vi "WSVCAP SHL FPGA LL Procedure RFFE - Send Data.vi"(0 "Procedure Step":T1, 1 "Wait Ticks Remaining":u32, 2 "CMD Length [1-48]":u8, 5 "RFFE Wait Ticks":u32, 7 "Write Bit Index [0-47]":u8, 9 "RFFE Cycle Mode":bool, 11 "error in (no error)":errorcluster, 12 "RFFE Cycle CMD":u64, 13 "Socket Mask":u64) -> (3 "Wait Ticks Remaining Out":u32, 4 "Procedure Step Out":T1, 8 "Write Bit Index [0-47] Out":u8, 10 "Finished":bool, 15 "error out":errorcluster)   [LabVIEW 2012]
uses:
  Type Defs/WSVCAP SHL Procedure Step Enum.ctl
  Type Defs/WSVCAP SHL RFFE Write Line Enum.ctl
  Type Defs/WSVCAP SHL FIFO Operation Enum.ctl
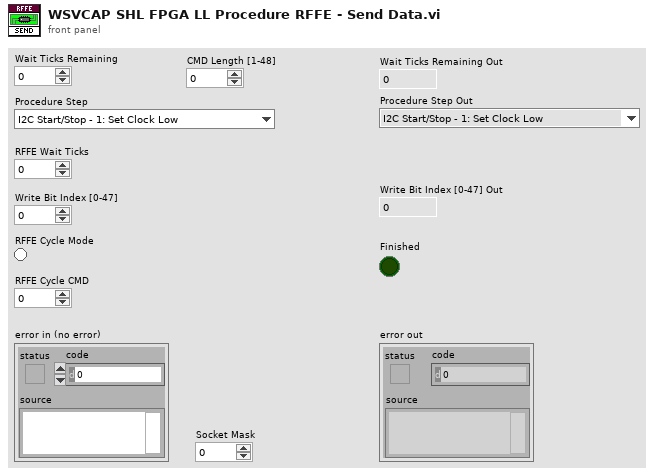
[diagram p1: front panel]
types:
  T1 = typedef "WSVCAP SHL Procedure Step Enum.ctl" = enum16{"I2C Start/Stop - 1: Set Clock Low", "I2C Start/Stop - 2: Wait", "I2C Start/Stop - 3: Set Data I", "I2C Start/Stop - 4: Wait", "I2C Start/Stop - 5: Set Clock High", "I2C Start/Stop - 6: Wait", "I2C Start/Stop - 7: Set Data II", "I2C Start/Stop - 8: Wait", "I2C Start/Stop - 9: Set Clock Low", "I2C Start/Stop - 10: Wait", "I2C Read ACK - 1: Set Clock High", "I2C Read ACK - 2: Wait", "I2C Read ACK - 3: Read ACK Bit", "I2C Read ACK - 4: Wait", "I2C Read ACK - 5: Set Clock Low", "I2C Read ACK - 6: Wait", "I2C Write ACK - 1: Write ACK Bit", "I2C Write ACK - 2: Wait", "I2C Write ACK - 3: Set Clock High", "I2C Write ACK - 4: Wait", "I2C Write ACK - 5: Set Clock Low", "I2C Write ACK - 6: Wait", "I2C Write ACK - 7: Set Data Low", "I2C Send Add - 1: Reset Bits Remaining", "I2C Send Add - 2: Set Data Bit", "I2C Send Add - 3: Wait", "I2C Send Add - 4: Set Clock High", "I2C Send Add - 5: Wait", "I2C Send Add - 6: Set Clock Low", "I2C Send Add - 7: Wait", "I2C Send Add - 8: Check Bits Remaining", "I2C Send Data - 1: Reset Bits Remaining", "I2C Send Data - 2: Load Write Bit from FIFO", "I2C Send Data - 3: Set Data Bit", "I2C Send Data - 4: Wait", "I2C Send Data - 5: Set Clock High", "I2C Send Data - 6: Wait", "I2C Send Data - 7: Set Clock Low", "I2C Send Data - 8: Wait", "I2C Send Data - 9: Check Bits Remaining", "I2C Receive Data - 1: Reset Bits Remaining", "I2C Receive Data - 2: Wait", "I2C Receive Data - 3: Set Clock High", "I2C Receive Data - 4: Wait", "I2C Receive Data - 5: Read Data Bit", "I2C Receive Data - 6: Wait", "I2C Receive Data - 7: Set Clock Low", "I2C Receive Data - 8: Wait", "I2C Receive Data - 9: Check Bits Remaining", "SPI Clear Lines - 1:Clear", "SPI Send/Receive - 1: Load SDA - Clock Low", "SPI Send/Receive - 2: Wait", "SPI Send/Receive - 3: Load DATO - Clock High", "SPI Send/Receive - 4: Wait", "SPI Wait CMD Delay - 1:Wait", "RFFE Send SSC - 1:Set Low", "RFFE Send SSC - 2:Wait", "RFFE Send SSC - 3:Set SDA High", "RFFE Send SSC - 4:Wait", "RFFE Send SSC - 5:Set SDA Low", "RFFE Send SSC - 6:Wait", "RFFE Send Data - 1:Set SCL High", "RFFE Send Data - 2:Wait", "RFFE Send Data - 3:Set SCL Low", "RFFE Send Data - 4:Wait", "RFFE Send Data - 5:Set SCL High (P)", "RFFE Send Data - 6:Wait", "RFFE Send Data - 7:Set SCL Low (P)", "RFFE Send Data - 8:Wait", "RFFE Send Data - 9:Set SCL High (BP)", "RFFE Send Data - 10:Wait", "RFFE Send Data - 11:Set SCL Low (BP)", "RFFE Send Data - 12:Wait", "RFFE Receive Data - 1:Set SCL High", "RFFE Receive Data - 2:Wait", "RFFE Receive Data - 3:Set SCL Low", "RFFE Receive Data - 4:Wait", "RFFE Receive Data - 5:Set SCL High (BP)", "RFFE Receive Data - 6:Wait", "RFFE Receive Data - 7:Set SCL Low (BP)", "RFFE Receive Data - 8:Wait", "RFFE Wait CMD Delay - 1:Wait", "RFFE Clear Lines - 1:Clear"}
  T2 = typedef "WSVCAP SHL RFFE Write Line Enum.ctl" = enum16{"SDAA", "SCLK"}
  T3 = typedef "WSVCAP SHL FIFO Operation Enum.ctl" = enum16{"Create FIFO/Memory", "Get Write FIFO Status", "Get Read FIFO Status", "Put Element in Write", "Put Element in Read", "Get Element from Write", "Get Element from Read"}
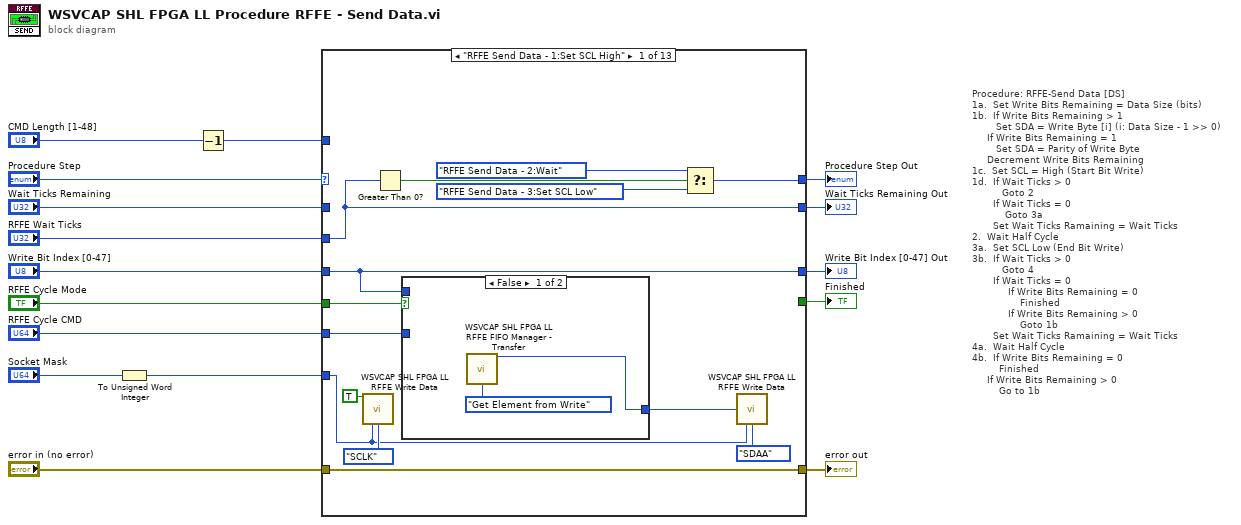
[diagram p0: block diagram]
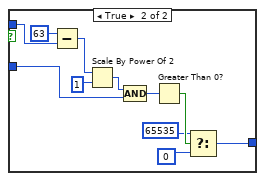
[diagram p2: hidden frame]
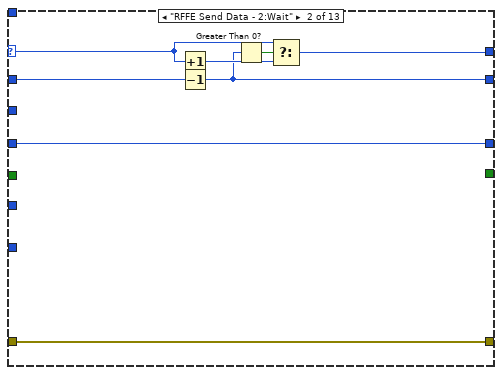
[diagram p3: hidden frame]
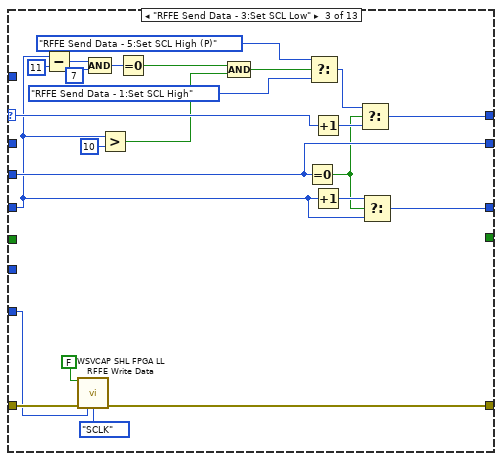
[diagram p4: hidden frame]
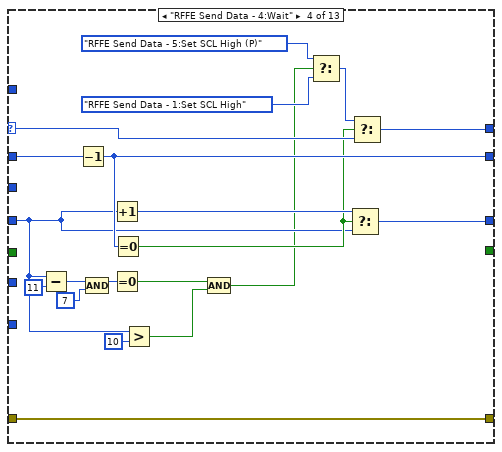
[diagram p5: hidden frame]
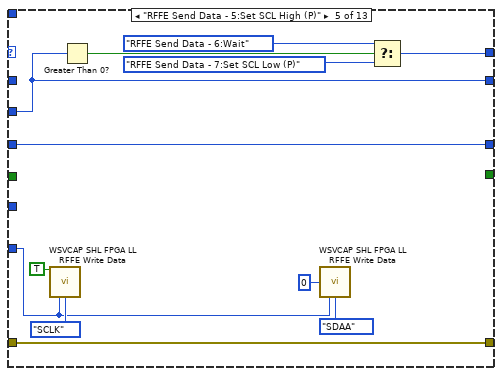
[diagram p6: hidden frame]
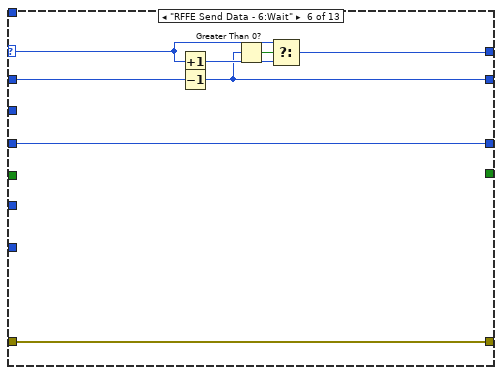
[diagram p7: hidden frame]
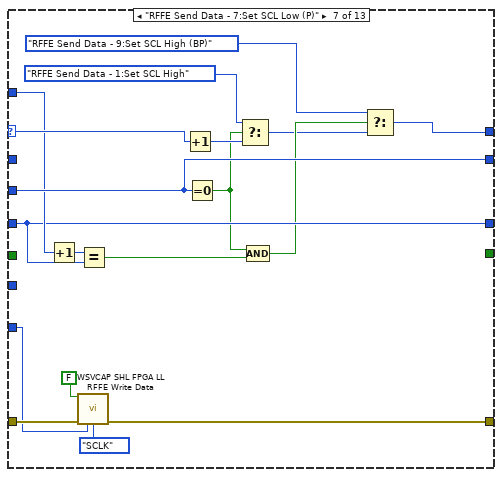
[diagram p8: hidden frame]
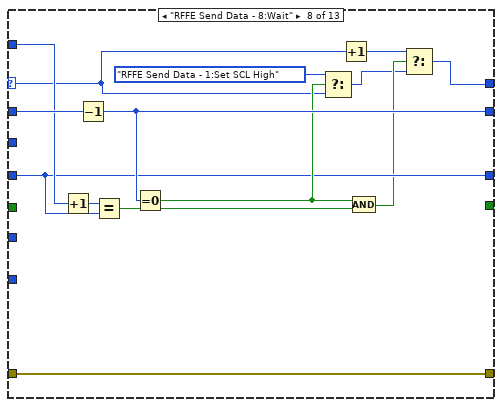
[diagram p9: hidden frame]
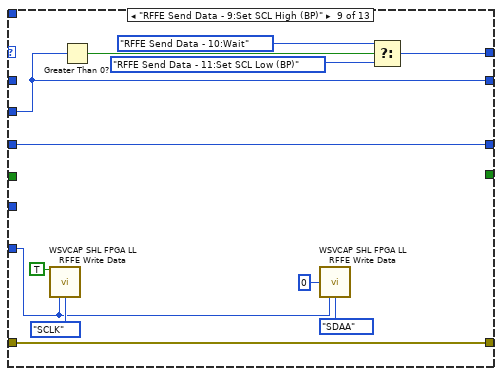
[diagram p10: hidden frame]
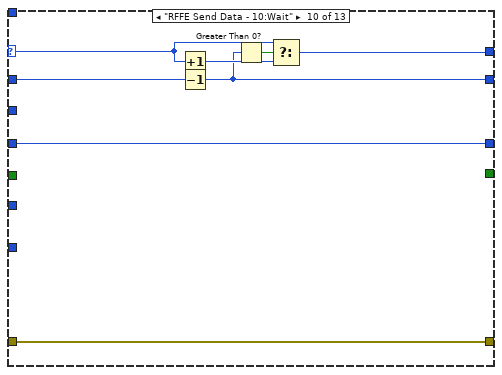
[diagram p11: hidden frame]
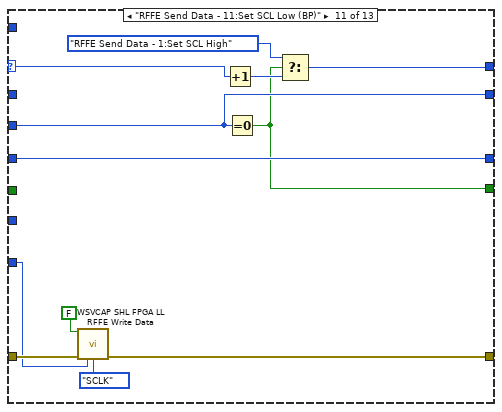
[diagram p12: hidden frame]
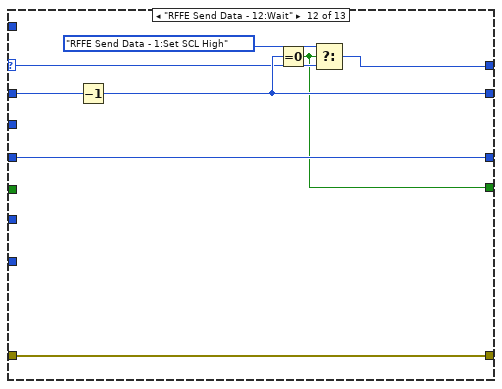
[diagram p13: hidden frame]
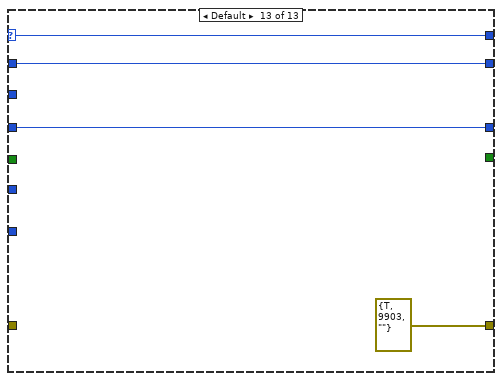
[diagram p14: hidden frame]
diagram:
  # "Procedure: RFFE-Send Data [DS]\n1a.  Set Write Bits Remaining = Data Size (bits)\n1b.  If Write Bits Remaining > 1\n        Set SDA = Write Byte [i] (i: Data Size - 1 >> 0)\n     If Write Bits Remaining = 1\n        Set SDA = Parity of Write Byte\n     Decrement Write Bits Remaining\n1c.  Set SCL = High (Start Bit Write)\n1d.  If Wait Ticks > 0\n          Goto 2\n       If Wait Ticks = 0 \n           Goto 3a\n       Set Wait Ticks Ramaining = Wait Ticks\n2.  Wait Half Cycle\n3a.  Set SCL Low (End Bit Write)\n3b.  If Wait Ticks > 0\n          Goto 4\n       If Wait Ticks = 0 \n            If Write Bits Remaining = 0\n                Finished\n            If Write Bits Remaining > 0\n                Goto 1b\n       Set Wait Ticks Ramaining = Wait Ticks\n4a.  Wait Half Cycle\n4b.  If Write Bits Remaining = 0\n         Finished\n     If Write Bits Remaining > 0\n         Go to 1b"
  n1 = To Unsigned Word Integer(number="Socket Mask") -> (unsigned 16bit integer=w12:u16)
  n2 = Decrement(x="CMD Length [1-48]") -> (x-1=w1:u8)
  n3 = case shown="\"RFFE Send Data - 1:Set SCL High\"" "Procedure Step" {
    selector: "Procedure Step" -> [_ w49 w75 w94 _ w113 w133 w136 _ w165 w179 w182 w190]
    tunnel: [w24 w51 w70 w95 w102 w115 w128 w147 w154 w167 w174 w187 errorcluster {"status"=TRUE, "code"=9903, "source"=""} ("error IO")] -> w15
    tunnel: "error in (no error)" -> [w24 w51 w71 w95 w102 w115 w129 w147 w154 w167 w175 w187 _]
    tunnel: "Wait Ticks Remaining" -> [_ w47 _ w93 _ w111 _ w146 _ w163 _ w186 w189]
    tunnel: "RFFE Wait Ticks" -> [w18 _ w66 _ w98 _ w126 _ w150 _ w171 _ _]
    tunnel: [_ _ _ _ _ _ _ _ _ _ w168 w180 _] -> w14
    tunnel: "Write Bit Index [0-47]" -> [w17 w44 w59 w82 w97 w108 w123 w141 w149 w160 w169 w183 w188]
    tunnel: w12 -> [w26 _ w69 _ w103 _ w127 _ w155 _ w173 _ _]
    tunnel: "RFFE Cycle Mode" -> [w23 _ _ _ _ _ _ _ _ _ _ _ _]
    tunnel: "RFFE Cycle CMD" -> [w22 _ _ _ _ _ _ _ _ _ _ _ _]
    tunnel: w1 -> [_ _ _ _ _ _ w124 w142 _ _ _ _ _]
    tunnel: [w19 w46 w67 w92 w99 w110 w116 w134 w151 w162 w172 w181 w190] -> w5
    tunnel: [w18 w45 w66 w91 w98 w109 w126 w145 w150 w161 w171 w185 w189] -> w4
    tunnel: [w17 w44 w65 w88 w97 w108 w123 w141 w149 w160 w169 w183 w188] -> w3
    frame "RFFE Send Data - 1:Set SCL High" {
      n4 = call "WSVCAP SHL FPGA LL RFFE Write Data.vi"("CLK In"=TRUE ("Bit In"), "Socket Mask"=w26, "Line"=WSVCAP_SHL_RFFE_Write_Line_Enum."SCLK") -> ()  [unwired: 12 in, 1 out]
      n5 = Greater Than 0?(x=w18) -> (x > 0?=w27:bool)
      n6 = case shown="False" w23 {
        tunnel: [w31 w37] -> w25
        tunnel: w22 -> [_ w36]
        tunnel: w17 -> [_ w34]
        frame False {
          n7 = call "WSVCAP SHL FPGA LL RFFE FIFO Manager - Transfer.vi"("Operation"=WSVCAP_SHL_FIFO_Operation_Enum."Get Element from Write") -> ("Data Out"=w31:u16)  [unwired: 12 in, 2 out]
        }
        frame True {
          n8 = Subtract(x=u8 63 ("y"), y=w34) -> (x-y=w33:u8)
          n9 = Scale By Power Of 2(n=w33, x=u64 1 ("Data Out")) -> (x*2^n=w42:u64)
          n10 = Compound Arithmetic op=AND(w42, w36) -> (w41:u64)
          n11 = Greater Than 0?(x=w41) -> (x > 0?=w40:bool)
          n12 = Select(t=u16 65535 ("Data Out"), s=w40, f=u16 0 ("Data Out")) -> (s? t:f=w37:u16)
        }
      }
      n13 = Select(t=WSVCAP_SHL_Procedure_Step_Enum."RFFE Send Data - 2:Wait" ("Procedure Step"), s=w27, f=WSVCAP_SHL_Procedure_Step_Enum."RFFE Send Data - 3:Set SCL Low" ("Procedure Step")) -> (s? t:f=w19:T1)
      n14 = call "WSVCAP SHL FPGA LL RFFE Write Data.vi"("Data Word In"=w25, "Socket Mask"=w26, "Line"=WSVCAP_SHL_RFFE_Write_Line_Enum."SDAA") -> ()  [unwired: 12 in, 1 out]
    }
    frame "RFFE Send Data - 2:Wait" {
      n15 = Increment(x=w49) -> (x+1=w48:T1)
      n16 = Decrement(x=w47) -> (x-1=w45:u32)
      n17 = Greater Than 0?(x=w45) -> (x > 0?=w50:bool)
      n18 = Select(t=w49, s=w50, f=w48) -> (s? t:f=w46:T1)
    }
    frame "RFFE Send Data - 3:Set SCL Low" {
      n19 = Subtract(x=w59, y=u8 11) -> (x-y=w54:u8)
      n20 = call "WSVCAP SHL FPGA LL RFFE Write Data.vi"("CLK In"=FALSE ("Bit In"), "error in (no error)"=w71, "Socket Mask"=w69, "Line"=WSVCAP_SHL_RFFE_Write_Line_Enum."SCLK") -> ("error out"=w70:errorcluster)  [unwired: 11 in]
      n21 = Compound Arithmetic op=AND(w54, u8 7 ("y")) -> (w52:u8)
      n22 = Greater?(x=w59, y=u8 10) -> (0:w56:bool)
      n23 = Equal To 0?(x=w52) -> (x = 0?=w57:bool)
      n24 = Compound Arithmetic op=AND(w57, w56) -> (w55:bool)
      n25 = Equal To 0?(x=w66) -> (x = 0?=w61:bool)
      n26 = Select(t=WSVCAP_SHL_Procedure_Step_Enum."RFFE Send Data - 5:Set SCL High (P)" ("Procedure Step"), s=w55, f=WSVCAP_SHL_Procedure_Step_Enum."RFFE Send Data - 1:Set SCL High" ("Procedure Step")) -> (s? t:f=w62:T1)
      n27 = Increment(x=w75) -> (x+1=w74:T1)
      n28 = Increment(x=w59) -> (x+1=w68:u8)
      n29 = Select(t=w62, s=w61, f=w74) -> (s? t:f=w67:T1)
      n30 = Select(t=w68, s=w61, f=w59) -> (s? t:f=w65:u8)
    }
    frame "RFFE Send Data - 4:Wait" {
      n31 = Subtract(x=w82, y=u8 11) -> (x-y=w78:u8)
      n32 = Decrement(x=w93) -> (x-1=w91:u32)
      n33 = Compound Arithmetic op=AND(w78, u8 7 ("y")) -> (w77:u8)
      n34 = Increment(x=w82) -> (x+1=w90:u8)
      n35 = Equal To 0?(x=w77) -> (x = 0?=w80:bool)
      n36 = Equal To 0?(x=w91) -> (x = 0?=w89:bool)
      n37 = Greater?(x=w82, y=u8 10) -> (0:w81:bool)
      n38 = Compound Arithmetic op=AND(w80, w81) -> (w79:bool)
      n39 = Select(t=WSVCAP_SHL_Procedure_Step_Enum."RFFE Send Data - 5:Set SCL High (P)" ("Procedure Step"), s=w79, f=WSVCAP_SHL_Procedure_Step_Enum."RFFE Send Data - 1:Set SCL High" ("Procedure Step")) -> (s? t:f=w85:T1)
      n40 = Select(t=w90, s=w89, f=w82) -> (s? t:f=w88:u8)
      n41 = Select(t=w85, s=w89, f=w94) -> (s? t:f=w92:T1)
    }
    frame "RFFE Send Data - 5:Set SCL High (P)" {
      n42 = call "WSVCAP SHL FPGA LL RFFE Write Data.vi"("CLK In"=TRUE ("Bit In"), "Socket Mask"=w103, "Line"=WSVCAP_SHL_RFFE_Write_Line_Enum."SCLK") -> ()  [unwired: 12 in, 1 out]
      n43 = Greater Than 0?(x=w98) -> (x > 0?=w104:bool)
      n44 = call "WSVCAP SHL FPGA LL RFFE Write Data.vi"("Data Word In"=u16 0, "Socket Mask"=w103, "Line"=WSVCAP_SHL_RFFE_Write_Line_Enum."SDAA") -> ()  [unwired: 12 in, 1 out]
      n45 = Select(t=WSVCAP_SHL_Procedure_Step_Enum."RFFE Send Data - 6:Wait" ("Procedure Step"), s=w104, f=WSVCAP_SHL_Procedure_Step_Enum."RFFE Send Data - 7:Set SCL Low (P)" ("Procedure Step")) -> (s? t:f=w99:T1)
    }
    frame "RFFE Send Data - 6:Wait" {
      n46 = Increment(x=w113) -> (x+1=w112:T1)
      n47 = Decrement(x=w111) -> (x-1=w109:u32)
      n48 = Greater Than 0?(x=w109) -> (x > 0?=w114:bool)
      n49 = Select(t=w113, s=w114, f=w112) -> (s? t:f=w110:T1)
    }
    frame "RFFE Send Data - 7:Set SCL Low (P)" {
      n50 = Increment(x=w124) -> (x+1=w120:u8)
      n51 = call "WSVCAP SHL FPGA LL RFFE Write Data.vi"("CLK In"=FALSE ("Bit In"), "error in (no error)"=w129, "Socket Mask"=w127, "Line"=WSVCAP_SHL_RFFE_Write_Line_Enum."SCLK") -> ("error out"=w128:errorcluster)  [unwired: 11 in]
      n52 = Equal?(x=w120, y=w123) -> (x = y?=w121:bool)
      n53 = Increment(x=w133) -> (x+1=w132:T1)
      n54 = Equal To 0?(x=w126) -> (x = 0?=w122:bool)
      n55 = Select(t=WSVCAP_SHL_Procedure_Step_Enum."RFFE Send Data - 1:Set SCL High" ("Procedure Step"), s=w122, f=w132) -> (s? t:f=w118:T1)
      n56 = Compound Arithmetic op=AND(w122, w121) -> (w119:bool)
      n57 = Select(t=WSVCAP_SHL_Procedure_Step_Enum."RFFE Send Data - 9:Set SCL High (BP)" ("Procedure Step"), s=w119, f=w118) -> (s? t:f=w116:T1)
    }
    frame "RFFE Send Data - 8:Wait" {
      n58 = Increment(x=w142) -> (x+1=w139:u8)
      n59 = Decrement(x=w146) -> (x-1=w145:u32)
      n60 = Equal?(x=w139, y=w141) -> (x = y?=w140:bool)
      n61 = Equal To 0?(x=w145) -> (x = 0?=w143:bool)
      n62 = Select(t=WSVCAP_SHL_Procedure_Step_Enum."RFFE Send Data - 1:Set SCL High" ("Procedure Step"), s=w143, f=w136) -> (s? t:f=w137:T1)
      n63 = Increment(x=w136) -> (x+1=w135:T1)
      n64 = Compound Arithmetic op=AND(w143, w140) -> (w138:bool)
      n65 = Select(t=w135, s=w138, f=w137) -> (s? t:f=w134:T1)
    }
    frame "RFFE Send Data - 9:Set SCL High (BP)" {
      n66 = call "WSVCAP SHL FPGA LL RFFE Write Data.vi"("CLK In"=TRUE ("Bit In"), "Socket Mask"=w155, "Line"=WSVCAP_SHL_RFFE_Write_Line_Enum."SCLK") -> ()  [unwired: 12 in, 1 out]
      n67 = Greater Than 0?(x=w150) -> (x > 0?=w156:bool)
      n68 = call "WSVCAP SHL FPGA LL RFFE Write Data.vi"("Data Word In"=u16 0, "Socket Mask"=w155, "Line"=WSVCAP_SHL_RFFE_Write_Line_Enum."SDAA") -> ()  [unwired: 12 in, 1 out]
      n69 = Select(t=WSVCAP_SHL_Procedure_Step_Enum."RFFE Send Data - 10:Wait" ("Procedure Step"), s=w156, f=WSVCAP_SHL_Procedure_Step_Enum."RFFE Send Data - 11:Set SCL Low (BP)" ("Procedure Step")) -> (s? t:f=w151:T1)
    }
    frame "RFFE Send Data - 10:Wait" {
      n70 = Increment(x=w165) -> (x+1=w164:T1)
      n71 = Decrement(x=w163) -> (x-1=w161:u32)
      n72 = Greater Than 0?(x=w161) -> (x > 0?=w166:bool)
      n73 = Select(t=w165, s=w166, f=w164) -> (s? t:f=w162:T1)
    }
    frame "RFFE Send Data - 11:Set SCL Low (BP)" {
      n74 = call "WSVCAP SHL FPGA LL RFFE Write Data.vi"("CLK In"=FALSE ("Bit In"), "error in (no error)"=w175, "Socket Mask"=w173, "Line"=WSVCAP_SHL_RFFE_Write_Line_Enum."SCLK") -> ("error out"=w174:errorcluster)  [unwired: 11 in]
      n75 = Increment(x=w179) -> (x+1=w178:T1)
      n76 = Equal To 0?(x=w171) -> (x = 0?=w168:bool)
      n77 = Select(t=WSVCAP_SHL_Procedure_Step_Enum."RFFE Send Data - 1:Set SCL High" ("Procedure Step"), s=w168, f=w178) -> (s? t:f=w172:T1)
    }
    frame "RFFE Send Data - 12:Wait" {
      n78 = Decrement(x=w186) -> (x-1=w185:u32)
      n79 = Equal To 0?(x=w185) -> (x = 0?=w180:bool)
      n80 = Select(t=WSVCAP_SHL_Procedure_Step_Enum."RFFE Send Data - 1:Set SCL High" ("Procedure Step"), s=w180, f=w182) -> (s? t:f=w181:T1)
    }
    frame Default {
    }
  }
  "error out" <- w15
  "Finished" <- w14
  "Procedure Step Out" <- w5
  "Wait Ticks Remaining Out" <- w4
  "Write Bit Index [0-47] Out" <- w3
